vi "Run_Core.vi"(0 "Message Popup in":refnum<class "Statement.lvclass">, 11 "error in (no error)":errorcluster) -> (4 "Message Popup out":refnum<class "Statement.lvclass">, 6 "Return":variant, 15 "error out":errorcluster)   [LabVIEW 2019, in "Statement.lvclass"]
uses:
  Statement.lvclass
  C:/Users/Patrick/Documents/GitHub/LabVIEW-Script-Language/source code/LSL components/functions/functionsbase/functionbase.lvclass
  Statement.lvclass/Statement.ctl
  functionsbase/functionbase.lvclass/functionbase.ctl
  functionsbase/properties/Read RT Variables.vi
  functionsbase/properties/Read Indent#.vi
  variables/RT Variables/RT Variables.lvclass
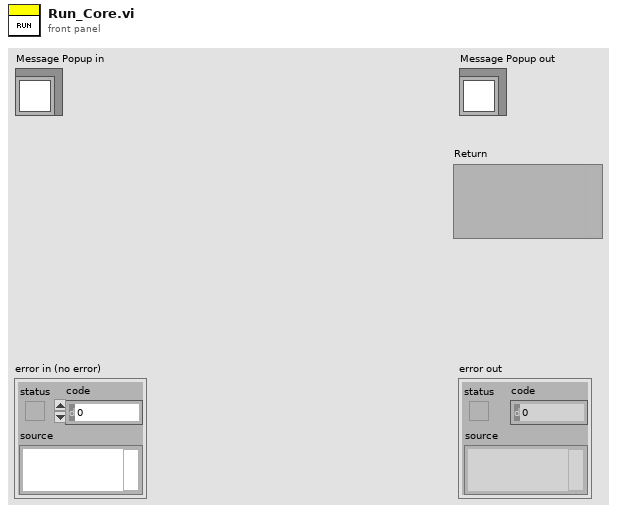
[diagram p1: front panel]
types:
  T1 = typedef "Statement.lvclass/Function List.ctl" = enum16{"Assignment Statement", "Comma Statement", "Unary Increament", "Unary Decrement"}
  T2 = typedef "Datatype.ctl" = enum16{"Null", "Numeric", "String", "Bool", "Numeric 1D", "String 1D", "Bool 1D", "Numeric 2D", "String 2D", "Bool 2D", "Variant"}
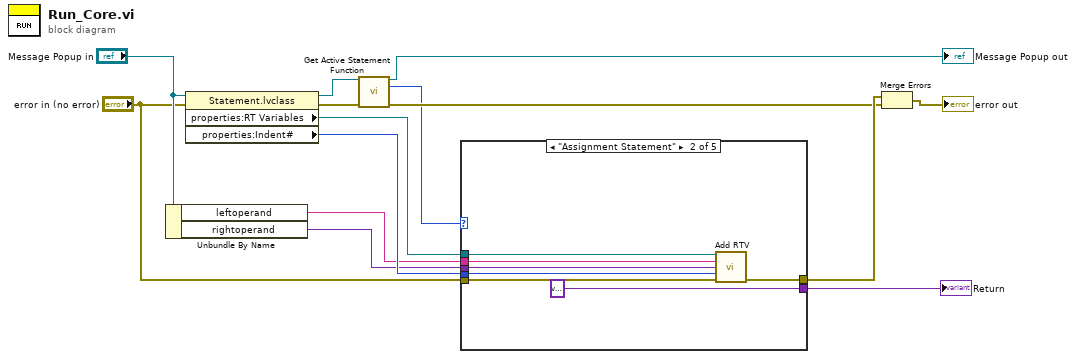
[diagram p0: block diagram]
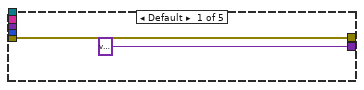
[diagram p2: hidden frame]
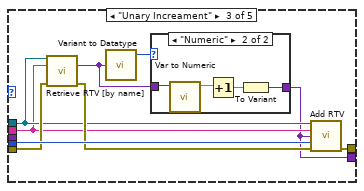
[diagram p3: hidden frame]
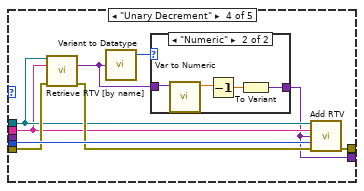
[diagram p5: hidden frame]
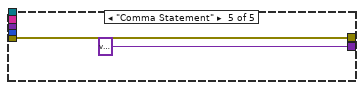
[diagram p7: hidden frame]
diagram:
  n1 = Unbundle By Name("Message Popup in") -> ("leftoperand"=w8:string, "rightoperand"=w9:variant)
  n2 = property class="Statement.lvclass"(reference="Message Popup in", error in="error in (no error)") -> (reference out=w4:refnum<class "Statement.lvclass">, error out=w6:errorcluster, "properties:RT Variables"=w10:refnum<class "RT Variables.lvclass">, "properties:Indent#"=w11:i64)
  n3 = call "Get Active Statement Function.vi"("Statement in"=w4, "error in (no error)"=w6) -> ("Statement out"=→"Message Popup out":refnum<class "Statement.lvclass">, "Function List"=w2:T1, "error out"=w5:errorcluster)  [unwired: 11 in]
  n4 = case shown="\"Assignment Statement\"" w2 {
    tunnel: "error in (no error)" -> [w16 w23 w30 w44 w53]
    tunnel: w11 -> [_ w22 w32 w46 _]
    tunnel: w10 -> [_ w21 w28 w42 _]
    tunnel: w9 -> [_ w20 _ _ _]
    tunnel: w8 -> [_ w19 w27 w41 _]
    tunnel: [w16 w18 w31 w45 w53] -> w7
    tunnel: [variant ("lefttocomma") variant ("lefttocomma") w24 w38 variant ("lefttocomma")] -> w1
    frame Default {
    }
    frame "Assignment Statement" {
      n5 = call-dynamic "Add RTV.vi"("RT Variables in"=w21, "RTV name"=w19, "Data"=w20, "Scope"=w22, "error in (no error)"=w23) -> ("error out"=w18:errorcluster)  [unwired: 9 in, 1 out]
    }
    frame "Unary Increament" {
      n6 = call-dynamic "Retrieve RTV [by name].vi"("RT Variables in"=w28, "RTV name"=w27, "error in (no error)"=w30) -> ("Data"=w25:variant, "error out"=w29:errorcluster)  [unwired: 8 in, 3 out]
      n7 = call "Variant to Datatype.vi"("Variant"=w25) -> ("Datatype"=w26:T2)  [unwired: 2 in, 2 out]
      n8 = case shown="\"Numeric\"" w26 {
        tunnel: w25 -> [w33 w37]
        tunnel: [w33 w34] -> w24
        frame "Null", Default {
        }
        frame "Numeric" {
          n9 = call "Var to Numeric.vi"("Variant"=w37) -> ("Numeric"=w36:dbl)  [unwired: 10 in]
          n10 = Increment(x=w36) -> (x+1=w35:dbl)
          n11 = To Variant(anything=w35) -> (Variant=w34:variant)
        }
      }
      n12 = call-dynamic "Add RTV.vi"("RT Variables in"=w28, "RTV name"=w27, "Data"=w24, "Scope"=w32, "error in (no error)"=w29) -> ("error out"=w31:errorcluster)  [unwired: 9 in, 1 out]
    }
    frame "Unary Decrement" {
      n13 = call-dynamic "Retrieve RTV [by name].vi"("RT Variables in"=w42, "RTV name"=w41, "error in (no error)"=w44) -> ("Data"=w39:variant, "error out"=w43:errorcluster)  [unwired: 8 in, 3 out]
      n14 = call "Variant to Datatype.vi"("Variant"=w39) -> ("Datatype"=w40:T2)  [unwired: 2 in, 2 out]
      n15 = case shown="\"Numeric\"" w40 {
        tunnel: w39 -> [w47 w51]
        tunnel: [w47 w48] -> w38
        frame "Null", Default {
        }
        frame "Numeric" {
          n16 = call "Var to Numeric.vi"("Variant"=w51) -> ("Numeric"=w50:dbl)  [unwired: 10 in]
          n17 = Decrement(x=w50) -> (x-1=w49:dbl)
          n18 = To Variant(anything=w49) -> (Variant=w48:variant)
        }
      }
      n19 = call-dynamic "Add RTV.vi"("RT Variables in"=w42, "RTV name"=w41, "Data"=w38, "Scope"=w46, "error in (no error)"=w43) -> ("error out"=w45:errorcluster)  [unwired: 9 in, 1 out]
    }
    frame "Comma Statement" {
    }
  }
  "Return" <- w1
  n20 = Merge Errors(w7, w5) -> (→"error out":errorcluster)
